vi "gen_data_paths_from_list.vi"(5 "Data index":i32[](array[numeric]), 7 "Item Names":string[](array[string]), 8 "error in (no error)":errorcluster, 11 "Folder path":path) -> (0 "error out":errorcluster, 3 "Array path":path[](array[path]))   [LabVIEW 2021]
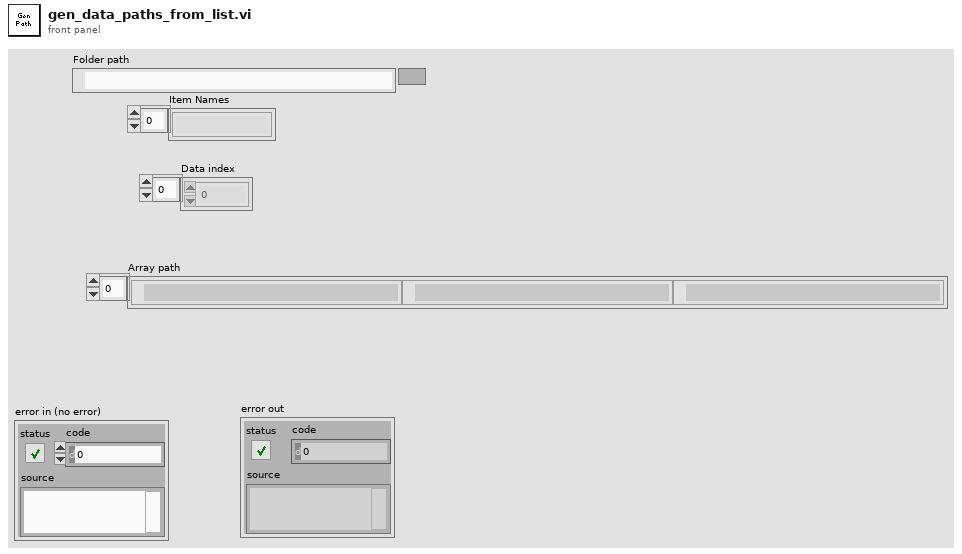
[diagram p1: front panel]
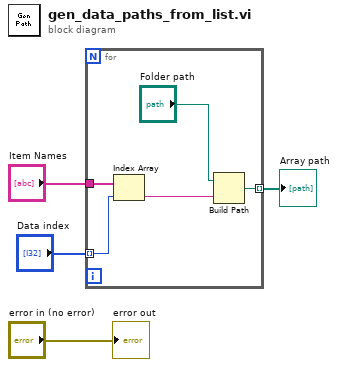
[diagram p0: block diagram]
diagram:
  n1 = for {
    tunnel: "Data index" -> [w9] mode=indexing
    tunnel: "Item Names" -> [w8]
    tunnel: [w5] -> w3 mode=indexing
    n2 = Index Array(array=w8, index=w9) -> (element=w6:string)
    n3 = Build Path(base path="Folder path", name or relative path=w6) -> (appended path=w5:path)
  }
  "Array path" <- w3
  "error out" <- "error in (no error)"
